vi "Square Root.vi"(0 "ABC":dbl[](array[numeric]), 5 "error in (no error)":errorcluster) -> (14 "Root":dbl[](array[numeric]), 19 "error out":errorcluster)   [LabVIEW 2013, in "Math.lvclass"]
uses:
  Math.lvclass
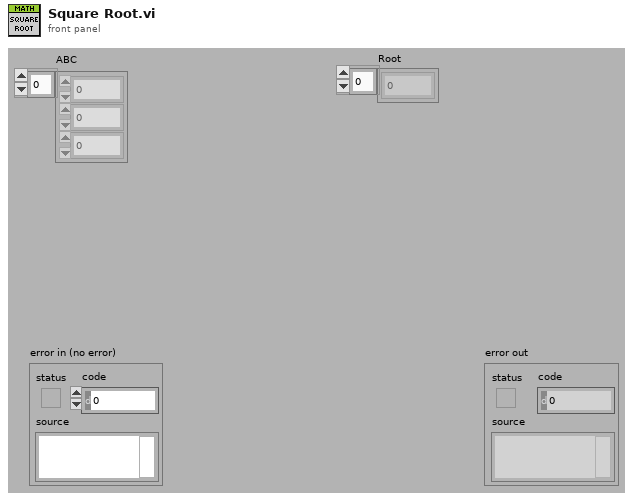
[diagram p1: front panel]
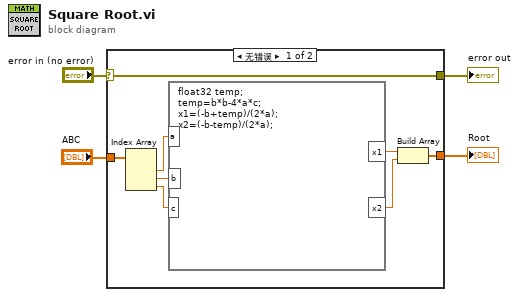
[diagram p0: block diagram]
diagram:
  n1 = case shown="无错误" "error in (no error)" {
    selector: "error in (no error)" -> [w12 w13]
    tunnel: [w12 w13] -> w3
    tunnel: "ABC" -> [w11 _]
    tunnel: [w5 _] -> w1
    frame No Error {
      n2 = Index Array(array=w11) -> (element #1=w10:dbl, element #2=w9:dbl, element #3=w8:dbl)  [unwired: 3 in]
      n3 = formula code="float32 temp;\ntemp=b*b-4*a*c;\nx1=(-b+temp)/(2*a);\nx2=(-b-temp)/(2*a);" ("公式节点")("a"=w10, "b"=w9, "c"=w8) -> ("x1"=w7:dbl, "x2"=w6:dbl)
      n4 = Build Array(w7, w6) -> (w5:dbl[])
    }
    frame Error {
    }
  }
  "error out" <- w3
  "Root" <- w1
